vi "sub_ubx-packet-analyzer.vi"(7 "cmd":enum16{"ubx str", "ubx u8arr"}(ring), 9 "ubx raw-u8arr":u8[](array[numeric]), 10 "start index":i32, 11 "ubx raw-str":string) -> (2 "val":bool, 3 "output":T1)   [LabVIEW 2019]
uses:
  Ctrl/ubx-packet.ctl
panel:
  out "CK_B":u8 format="%02x"
  out "CK_A":u8 format="%02x"
  out "chksum pk":u8[](array[numeric]) format="%02x"
  out "sync char":u8[](array[numeric]) format="%x"
  out "msg id":u8 format="%02x"
  out "msg class":u8 format="%02x"
  out "chksum":u8[](array[numeric]) format="%02x"
  out "payload":u8[](array[numeric]) format="%02x"
  out "next":u8[](array[numeric]) format="%02x"
  out "x+y":i32
  out "len":u8
  out "len_raw":i32
  out "start index":i32
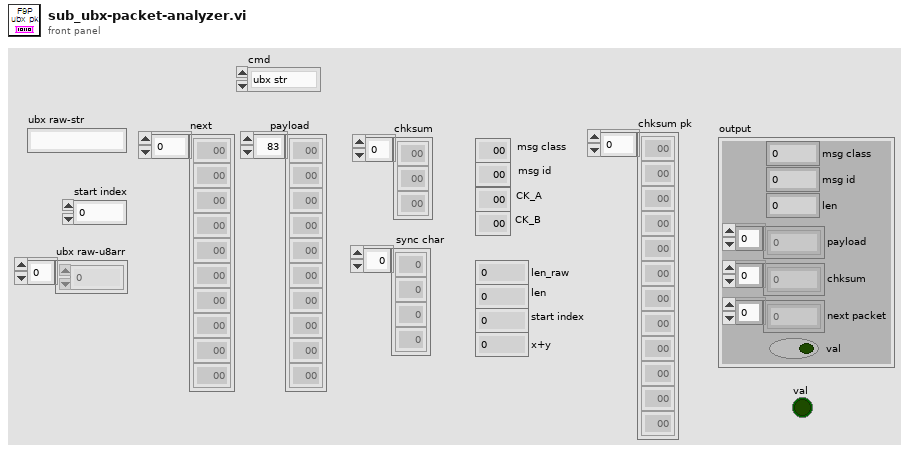
[diagram p1: front panel]
types:
  T1 = typedef "ubx-packet.ctl" = cluster{"msg class":u8, "msg id":u8, "len":u8, "payload":u8[], "chksum":u8[], "next packet":u8[], "val":bool}
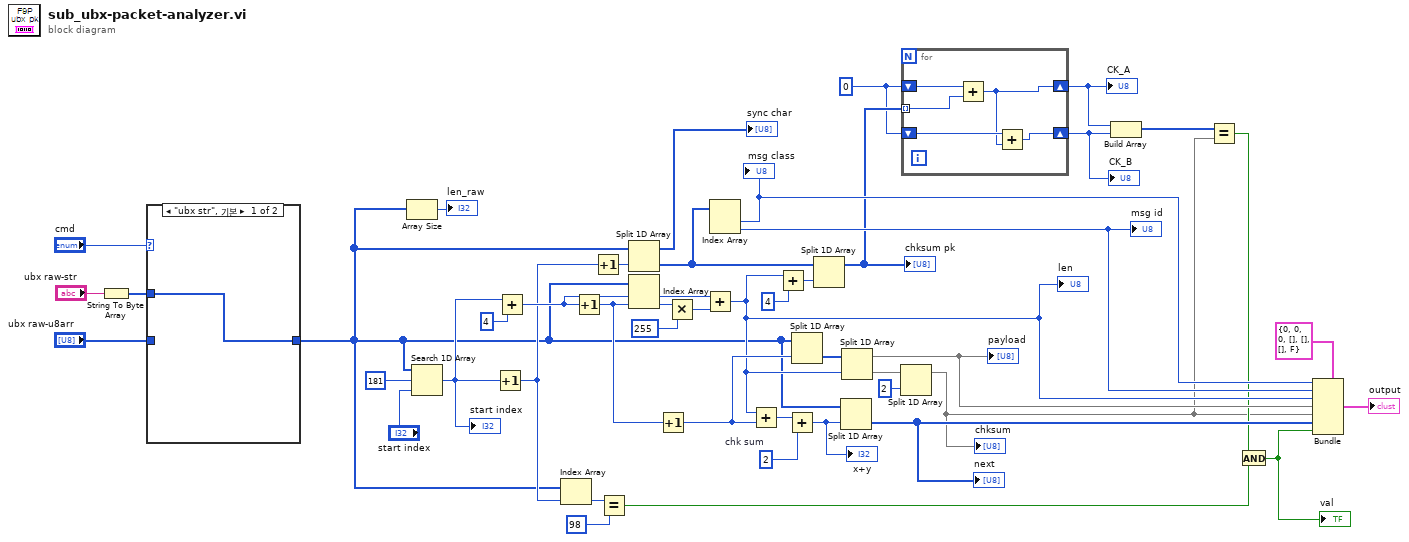
[diagram p0: block diagram]
diagram:
  w15 = u8 0 ("y")
  w34 = 2  # chk sum
  n1 = String To Byte Array(string="ubx raw-str") -> (unsigned byte array=w3:u8[])
  n2 = case shown="\"ubx str\", 기본" "cmd" {
    tunnel: w3 -> [w48 _]
    tunnel: "ubx raw-u8arr" -> [_ w49]
    tunnel: [w48 w49] -> w1
    frame "ubx str", Default {
    }
    frame "ubx u8arr" {
    }
  }
  n3 = Array Size(array=w1) -> (size(s)=→"len_raw":i32)
  n4 = Search 1D Array(1D array=w1, element=u8 181 ("원소"), start index (0)="start index") -> (index of element=w38:i32)
  "start index" <- w38
  n5 = Increment(x=w38) -> (x+1=w25:i32)
  n6 = Add(x=w38, y=4 ("인덱스")) -> (x+y=w36:i32)
  n7 = Index Array(array=w1, index=w25) -> (element=w41:u8)
  n8 = Increment(x=w36) -> (x+1=w32:i32)
  n9 = Increment(x=w25) -> (x+1=w23:i32)
  n10 = Equal?(x=w41, y=u8 98) -> (x = y?=w10:bool)
  n11 = Split 1D Array(array=w1, index=w23) -> (first subarray=→"sync char":u8[], second subarray=w20:u8[])
  n12 = Index Array(array=w1, index #1=w36, index #2=w32) -> (element #1=w42:u8, element #2=w45:u8)
  n13 = Increment(x=w32) -> (x+1=w31:i32)
  n14 = Multiply(x=w45, y=u8 255) -> (x*y=w43:u8)
  n15 = Add(x=w42, y=w43) -> (x+y=w18:u8)
  "len" <- w18
  n16 = Index Array(array=w20) -> (element #1=w24:u8, element #2=w21:u8)  [unwired: 2 in]
  "msg class" <- w24
  "msg id" <- w21
  n17 = Add(x=w18, y=w31) -> (x+y=w35:i32)
  n18 = Add(x=w18, y=u8 4) -> (x+y=w19:u8)
  n19 = Add(x=w35, y=w34) -> (x+y=w33:i32)
  "x+y" <- w33
  n20 = Split 1D Array(array=w1, index=w31) -> (second subarray=w30:u8[])  [unwired: 1 out]
  n21 = Split 1D Array(array=w20, index=w19) -> (first subarray=w16:u8[])  [unwired: 1 out]
  "chksum pk" <- w16
  n22 = Split 1D Array(array=w1, index=w33) -> (second subarray=w26:u8[])  [unwired: 1 out]
  "next" <- w26
  n23 = Split 1D Array(array=w30, index=w18) -> (first subarray=w27:u8[], second subarray=w29:u8[])
  "payload" <- w27
  n24 = Split 1D Array(array=w29, index=2 ("인덱스")) -> (first subarray=w8:u8[])  [unwired: 1 out]
  "chksum" <- w8
  n25 = for {
    tunnel: w16 -> [w54] mode=indexing
    shift-right: [w51] -> w14
    shift-left: w15 -> [w53]
    shift-right: [w50] -> w13
    shift-left: w15 -> [w52]
    n26 = Add(x=w53, y=w54) -> (x+y=w51:u8)
    n27 = Add(x=w52, y=w51) -> (x+y=w50:u8)
  }
  "CK_A" <- w14
  "CK_B" <- w13
  n28 = Build Array(w14, w13) -> (w12:u8[])
  n29 = Equal?(x=w12, y=w8) -> (x = y?=w11:bool)
  n30 = And(x=w11, y=w10) -> (x .and. y?=w9:bool)
  "val" <- w9
  n31 = Bundle(cluster=T1 {"msg class"=0, "msg id"=0, "len"=0, "payload"=[], "chksum"=[], "next packet"=[], "val"=FALSE} ("UBX packet"), "msg class"=w24, "msg id"=w21, "len"=w18, "payload"=w27, "chksum"=w8, "next packet"=w26, "val"=w9) -> (→"output":T1)
